vi "anda_ate_tocar.vi"() -> ()   [LabVIEW 2016]
uses:
  <vilib>/NXT/Subs/LVHSConnector.ctl
  <vilib>/NXT/LegoClasses/BrickReference/BrickReference.lvclass
  <vilib>/NXT/Block Support/NXT_OutputPort.ctl
  <vilib>/NXT/Block Support/NXT_InputPort.ctl
  <vilib>/NXT/Dual Mode Library/Motors/ResetMotor.vi
  <vilib>/NXT/Dual Mode Library/Motors/Rotation.vi
  <vilib>/NXT/Dual Mode Library/Sensors/Touch_Pressed.vi
  <vilib>/NXT/Dual Mode Library/Display/drawNumber.vi
  <vilib>/NXT/NXTIO Xnodes/AddressXNode/NXTIOAddress.xnode
panel:
  out "Angle of Rotation":i32
  in  "NXT/EV3":T1
  out "NXT/EV3 2":T1
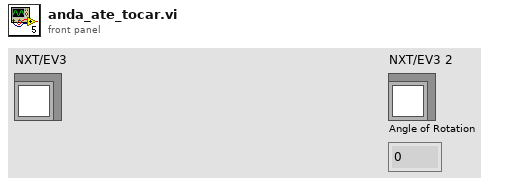
[diagram p1: front panel]
types:
  T1 = typedef "LVHSConnector.ctl" = refnum<class "BrickReference.lvclass">
  T2 = typedef "NXT_OutputPort.ctl" = u8
  T3 = typedef "NXT_InputPort.ctl" = u32
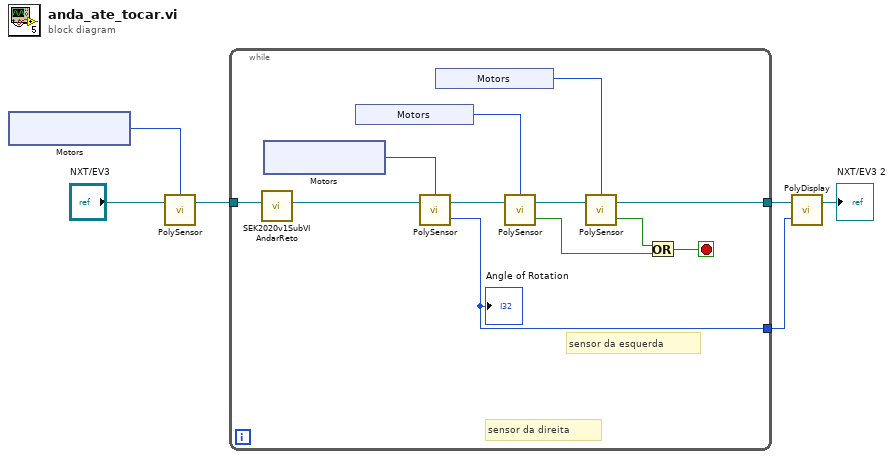
[diagram p0: block diagram]
diagram:
  n1 = xnode "Motors"() -> ("Motor"=w2:T2)
  n2 = call-poly <vilib>:"PolySensor.vi"("NXT/EV3"="NXT/EV3", "Port (All Ports)"=w2) -> ("NXT/EV3"=w1:T1)  [unwired: 2 out]
  n3 = while {
    tunnel: w1 -> [w9]
    tunnel: [w10] -> w4
    tunnel: [w18] -> w5
    stop <- w12 stop-if-true
    # "sensor da esquerda"
    # "sensor da direita"
    n4 = call "SEK2020v1SubVIAndarReto.vi"("NXT/EV3"=w9) -> ("NXT/EV3 2"=w8:T1)  [unwired: 9 in]
    n5 = xnode "Motors"() -> ("Motor"=w7:T2)
    n6 = xnode "Motors"() -> ("Sensor"=w16:T3)
    n7 = call-poly <vilib>:"PolySensor.vi"("NXT/EV3"=w8, "Port (Port A)"=w7) -> ("Angle of Rotation"=w18:i32, "NXT/EV3"=w11:T1)  [unwired: 1 out]
    "Angle of Rotation" <- w18
    n8 = xnode "Motors"() -> ("Sensor"=w15:T3)
    n9 = call-poly <vilib>:"PolySensor.vi"("NXT/EV3"=w11, "Port (Port 1)"=w16) -> ("Yes / No"=w13:bool, "NXT/EV3"=w17:T1)  [unwired: 1 in]
    n10 = call-poly <vilib>:"PolySensor.vi"("NXT/EV3"=w17, "Port (Port 1)"=w15) -> ("Yes / No"=w14:bool, "NXT/EV3"=w10:T1)  [unwired: 1 in]
    n11 = Or(x=w14, y=w13) -> (x .or. y?=w12:bool)
  }
  n12 = call-poly <vilib>:"PolyDisplay.vi"("number"=w5, "NXT/EV3"=w4) -> ("NXT/EV3"=→"NXT/EV3 2":T1)  [unwired: 2 in]
